vi "DB Operation.vi"(0 "connection reference":T1, 1 "DB Op Selector":T2, 2 "data":variant, 3 "Condition":string, 5 "table":string, 7 "columns":string[](array[string]), 9 "SQL Query":string, 11 "error in (no error)":errorcluster) -> (4 "connection reference out":T1, 8 "data out":variant[][](array[variant]), 15 "error out":errorcluster)   [LabVIEW 2024]
uses:
  CTRLS/DB operation Selector.ctl
  <vilib>/addons/database/Connection.llb/Conn ObjectReference.ctl
  <vilib>/addons/database/Connection.llb/Conn Execute.vi
  <vilib>/addons/database/Recordset.llb/Rec Fetch Recordset Data (R).vi
  <vilib>/addons/database/Recordset.llb/Rec Destroy - Connection.vi
  <vilib>/addons/database/NI_Database_API.lvlib
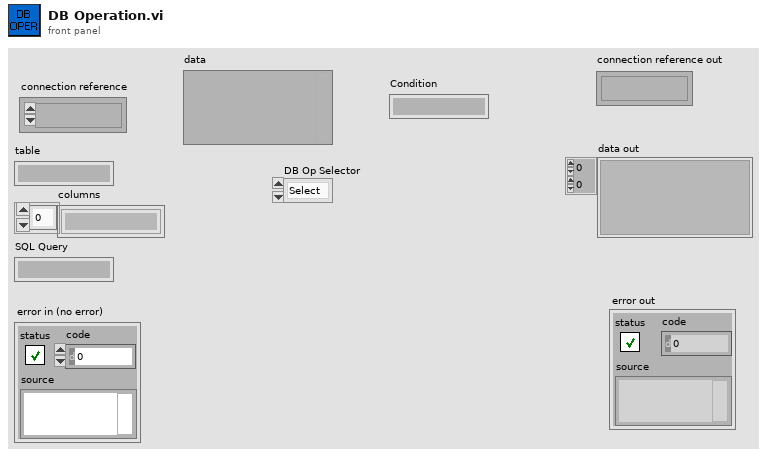
[diagram p1: front panel]
types:
  T1 = typedef "NI_Database_API.lvlib/Conn ObjectReference.ctl" = refnum<k1>
  T2 = typedef "DB operation Selector.ctl" = enum16{"Select", "Insert", "Update", "Execute select Query", "Execute update query"}
  T3 = typedef "NI_Database_API.lvlib/Rec ObjectReference.ctl" = refnum<k1>
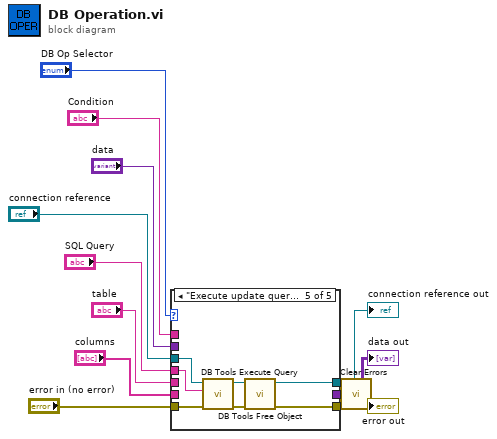
[diagram p0: block diagram]
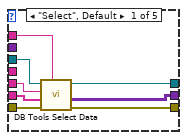
[diagram p2: hidden frame]
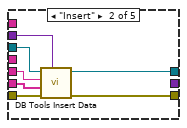
[diagram p3: hidden frame]
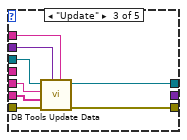
[diagram p4: hidden frame]
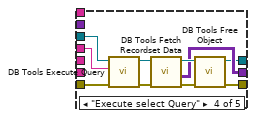
[diagram p5: hidden frame]
diagram:
  n1 = case shown="\"Execute update query\"" "DB Op Selector" {
    tunnel: "connection reference" -> [w20 w27 w35 w39 w51]
    tunnel: "data" -> [_ w26 w34 _ _]
    tunnel: "table" -> [w19 w25 w33 _ _]
    tunnel: "columns" -> [w18 w24 w32 _ _]
    tunnel: "error in (no error)" -> [w16 w23 w31 w41 w52]
    tunnel: [w15 w22 w30 w36 w48] -> w6
    tunnel: "Condition" -> [w17 _ w28 _ _]
    tunnel: [w14 _ _ w42 _] -> w4
    tunnel: [w13 w21 w29 w37 w49] -> w3
    tunnel: "SQL Query" -> [_ _ _ w38 w50]
    frame "Select", Default {
      n2 = call <vilib>:"DB Tools Select Data.vi"("condition"=w17, "error in (no error)"=w16, "columns"=w18, "table"=w19, "connection reference"=w20) -> ("error out"=w15:errorcluster, "data"=w14:variant[][], "connection reference out"=w13:T1)  [unwired: 1 in]
    }
    frame "Insert" {
      n3 = call <vilib>:"DB Tools Insert Data.vi"("data"=w26, "error in (no error)"=w23, "columns"=w24, "table"=w25, "connection reference"=w27) -> ("error out"=w22:errorcluster, "connection reference out"=w21:T1)  [unwired: 5 in]
    }
    frame "Update" {
      n4 = call <vilib>:"DB Tools Update Data.vi"("condition"=w28, "data"=w34, "error in (no error)"=w31, "columns"=w32, "table"=w33, "connection reference"=w35) -> ("error out"=w30:errorcluster, "connection reference out"=w29:T1)  [unwired: 4 in]
    }
    frame "Execute select Query" {
      n5 = call-poly <vilib>:"DB Tools Execute Query.vi"("error in (no error)"=w41, "SQL query"=w38, "connection reference"=w39) -> ("error out"=w40:errorcluster, "recordset reference"=w45:T3)  [unwired: 5 in]
      n6 = call-poly <vilib>:"DB Tools Fetch Recordset Data.vi"("error in (no error)"=w40, "recordset reference"=w45) -> ("error out"=w43:errorcluster, "recordset data"=w42:variant[][], "recordset reference out"=w44:T3)  [unwired: 3 in]
      n7 = call-poly <vilib>:"DB Tools Free Object.vi"("error in (no error)"=w43, "recordset reference"=w44) -> ("error out"=w36:errorcluster, "connection reference"=w37:T1)  [unwired: 8 in]
    }
    frame "Execute update query" {
      n8 = call-poly <vilib>:"DB Tools Execute Query.vi"("error in (no error)"=w52, "SQL query"=w50, "connection reference"=w51) -> ("error out"=w46:errorcluster, "recordset reference"=w47:T3)  [unwired: 5 in]
      n9 = call-poly <vilib>:"DB Tools Free Object.vi"("error in (no error)"=w46, "recordset reference"=w47) -> ("error out"=w48:errorcluster, "connection reference"=w49:T1)  [unwired: 8 in]
    }
  }
  "connection reference out" <- w3
  "data out" <- w4
  n10 = call <vilib>:"Clear Errors.vi"("error in (no error)"=w6) -> ("error out"=→"error out":errorcluster)  [unwired: 5 in, 1 out]
